vi "Partial.vi"() -> ()   [LabVIEW 2020, in "Examples.lvlib"]
uses:
  Examples.lvlib
  classes/Dual/Dual.lvclass/Dual.ctl
  <vilib>/Analysis/baseanly.llb/Dot Product.vi
  <vilib>/Analysis/baseanly.llb/Real Dot Product.vi
  <vilib>/Analysis/_algsub.llb/Vector Norm.vi
  <vilib>/Analysis/_algsub.llb/Real Vector Norm.vi
  Automatic Differentiation/Evaluate Gradient.vi
  Automatic Differentiation/Evaluate Partial Derivative.vi/49352e5e-86b6-4795-9dd0-b0f70ab2ee45.vi
  classes/Dual/Add infinitesimal to Double.vi
  classes/Dual/Read Dual Part.vi
  Automatic Differentiation/Evaluate Gradient.vi/3428a883-4abf-4854-9978-3fd53a24097c.vi
  Automatic Differentiation/Evaluate Partial Derivative.vi/49352e5e-86b6-4795-9dd0-b0f70ab2ee45.vi/5957e011-cf56-4527-b6ed-13c3a4ca997b.vi
  classes/Dual/Write a.vi
  Automatic Differentiation/Evaluate Gradient.vi/3428a883-4abf-4854-9978-3fd53a24097c.vi/5957e011-cf56-4527-b6ed-13c3a4ca997b.vi
  Multidimensional Test Function.vi
  classes/Dual/Dual.lvclass
  Automatic Differentiation/Automatic Differentiation.lvlib
panel:
  out "Grad_v f(x)":dbl format="%.2f"
  out "df(x_1,...,x_n)/dx_i":dbl
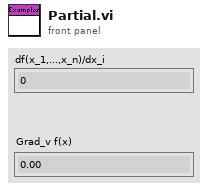
[diagram p1: front panel]
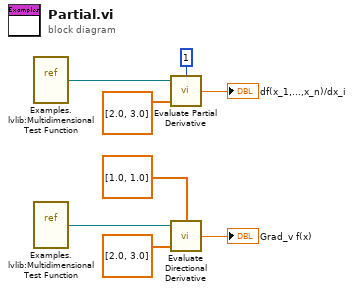
[diagram p0: block diagram]
diagram:
  n1 = vi-ref "Examples.lvlib:Multidimensional Test Function.vi"() -> (w5:refnum<vi>)
  n2 = vi-ref "Examples.lvlib:Multidimensional Test Function.vi"() -> (w4:refnum<vi>)
  n3 = call "Evaluate Partial Derivative.vi"("Partial Index"=1 ("Partial index"), "x=(x_1, ..., x_n)"=dbl[] [2.0, 3.0] ("(x_1,...,x_n)"), "Function Reference"=w5) -> ("df(x_1, ..., x_n)/dx_i"=→"df(x_1,...,x_n)/dx_i":dbl)  [unwired: 1 in]
  n4 = call "Evaluate Directional Derivative.vi"("Direction v=(v_1, ..., v_n)"=dbl[] [1.0, 1.0], "Point x=(x_1, ..., x_n)"=dbl[] [2.0, 3.0] ("(x_1,...,x_n)"), "Function Reference"=w4) -> ("Grad_v f(x)"=→"Grad_v f(x)":dbl)  [unwired: 1 in]
